vi "readConfig.vi"(8 "error in (no error)":errorcluster, 9 "config":string, 10 "deviceName":string, 11 "DDSFileReader in":refnum<class "DDSFileReader.lvclass">) -> (0 "error out":errorcluster, 3 "DDSFileReader out":refnum<class "DDSFileReader.lvclass">)   [LabVIEW 2011, in "Tools.lvlib" / "Filing.lvlib" / "DDSFileReader.lvclass"]
uses:
  DDSFileReader.lvclass
  DDSFileReader.lvclass/DDSFileReader.ctl
  FileReader.lvclass
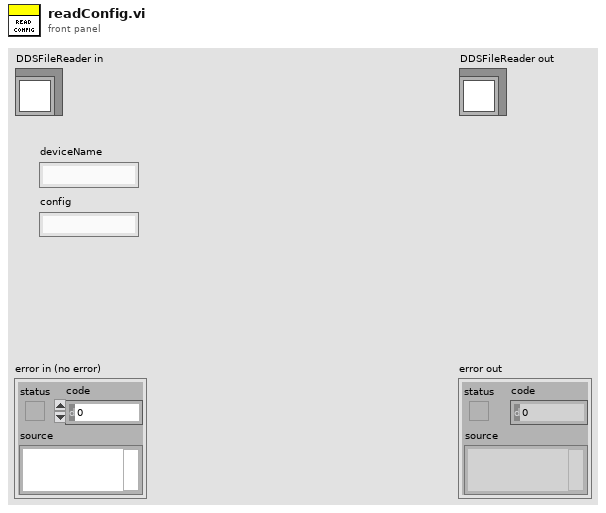
[diagram p1: front panel]
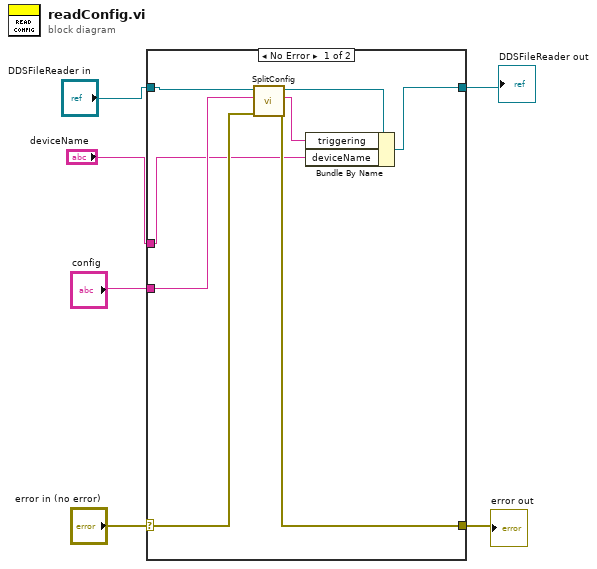
[diagram p0: block diagram]
diagram:
  n1 = case shown="No Error" "error in (no error)" {
    selector: "error in (no error)" -> [w13 w15]
    tunnel: "DDSFileReader in" -> [w14 w16]
    tunnel: [w9 w16] -> w2
    tunnel: [w8 w15] -> w1
    tunnel: "config" -> [w12 _]
    tunnel: "deviceName" -> [w7 _]
    frame No Error {
      n2 = call "SplitConfig.vi"("error in (no error)"=w13, "Config"=w12, "FileReader in"=w14) -> ("error out"=w8:errorcluster, "triggering"=w10:string, "FileReader out"=w11:refnum<class "DDSFileReader.lvclass">)  [unwired: 4 in, 2 out]
      n3 = Bundle By Name(cluster=w11, "triggering"=w10, "deviceName"=w7) -> (w9:refnum<class "DDSFileReader.lvclass">)
    }
    frame Error {
    }
  }
  "error out" <- w1
  "DDSFileReader out" <- w2
